vi "Cartesian to Cylindrical.vi"(4 "Cartesian\nCoordinates":cluster{"x":dbl, "y":dbl, "z":dbl}) -> (1 "Cylindrical\nCoordinates":cluster{"r":dbl, "theta":dbl, "z":dbl})   [LabVIEW 2013]
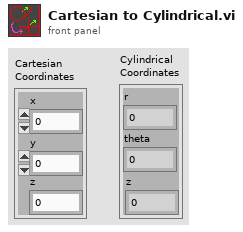
[diagram p1: front panel]
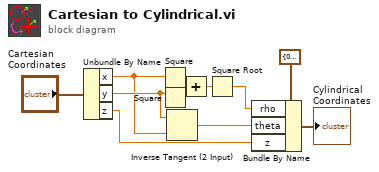
[diagram p0: block diagram]
diagram:
  n1 = Unbundle By Name("Cartesian\nCoordinates") -> ("x"=w3:dbl, "y"=w4:dbl, "z"=w1:dbl)
  n2 = Square(x=w3) -> (x^2=w6:dbl)
  n3 = Square(x=w4) -> (x^2=w7:dbl)
  n4 = Inverse Tangent (2 Input)(1:w3, 2:w4) -> (0:w2:dbl)
  n5 = Add(x=w6, y=w7) -> (x+y=w5:dbl)
  n6 = Square Root(x=w5) -> (sqrt(x)=w8:dbl)
  n7 = Bundle By Name(cluster=cluster{"rho":dbl, "theta":dbl, "z":dbl} {"rho"=0.0, "theta"=0.0, "z"=0.0} ("input cluster"), "rho"=w8, "theta"=w2, "z"=w1) -> (→"Cylindrical\nCoordinates":cluster{"rho":dbl, "theta":dbl, "z":dbl})
